vi "ExportPacketToCSV.vi"(6 "DefaultFolderName(Data)":string="Data", 7 "Prompt":string, 8 "Comment":string, 9 "NumerOfSamplesForAxis":i32, 10 "GyroData":waveform(dbl)[](array[waveform]), 11 "AccelData":waveform(dbl)[](array[waveform])) -> (0 "ErrorOut":errorcluster, 1 "Exported?":bool)   [LabVIEW 2016]
uses:
  <vilib>/Utility/file.llb/Write Delimited Spreadsheet (string).vi
  <vilib>/Utility/file.llb/Write Delimited Spreadsheet (DBL).vi
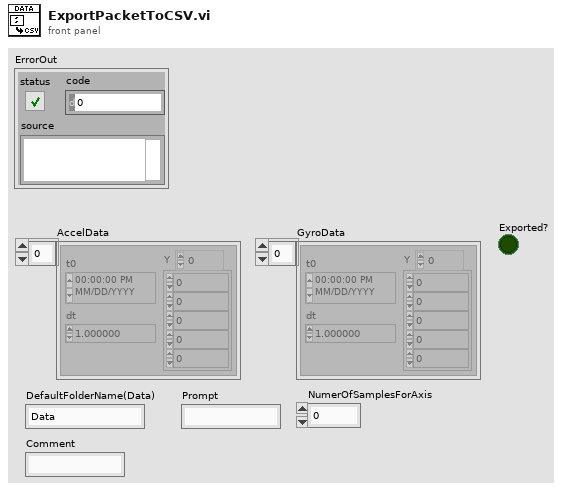
[diagram p1: front panel]
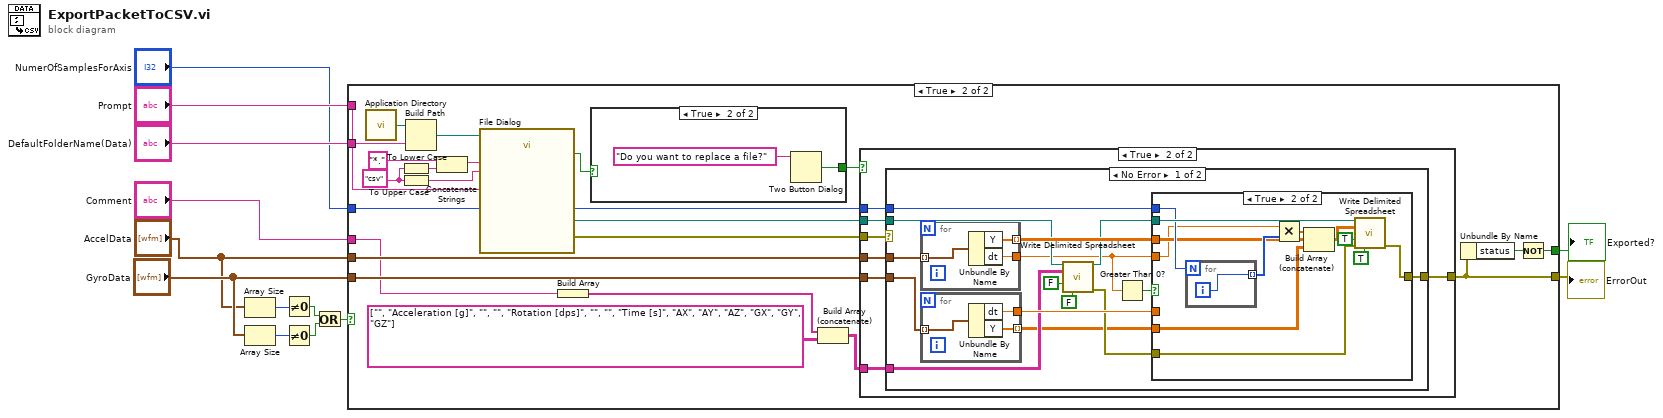
[diagram p0: block diagram]
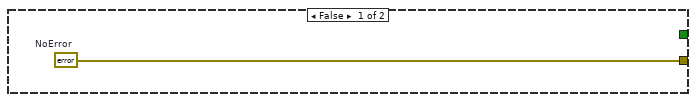
[diagram p2: hidden frame]
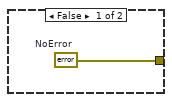
[diagram p3: hidden frame]
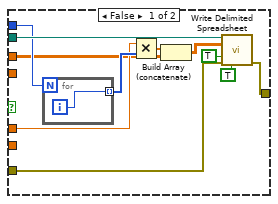
[diagram p4: hidden frame]
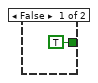
[diagram p6: hidden frame]
diagram:
  n1 = Array Size(array="AccelData") -> (size(s)=w8:i32)
  n2 = Array Size(array="GyroData") -> (size(s)=w9:i32)
  n3 = Not Equal To 0?(x=w8) -> (x != 0?=w6:bool)
  n4 = Not Equal To 0?(x=w9) -> (x != 0?=w5:bool)
  n5 = Or(x=w6, y=w5) -> (x .or. y?=w4:bool)
  n6 = case shown="True" w4 {
    tunnel: "DefaultFolderName(Data)" -> [_ w37]
    tunnel: [w14 w21] -> w12
    tunnel: "Prompt" -> [_ w36]
    tunnel: "GyroData" -> [_ w25]
    tunnel: "AccelData" -> [_ w24]
    tunnel: "NumerOfSamplesForAxis" -> [_ w22]
    tunnel: [_ w19] -> w2
    tunnel: "Comment" -> [_ w16]
    frame False {
      w14 = errorcluster {"status"=FALSE, "code"=0, "source"=""}  # NoError
    }
    frame True {
      w27 = "csv" ("string")
      n7 = call <vilib>:"Application Directory.vi"() -> ("Application Directory"=w35:path)
      n8 = To Lower Case(string=w27) -> (all lower case string=w32:string)
      n9 = To Upper Case(1:w27) -> (0:w33:string)
      n10 = Build Path(base path=w35, name or relative path=w37) -> (appended path=w34:path)
      n11 = Concatenate Strings("*." ("string"), w32) -> (w30:string)
      n12 = call "File Dialog"("start path"=w34, "prompt"=w36, "pattern (all files)"=w30, "pattern label"=w33) -> ("selected path"=w29:path, "exists"=w26:bool, "error out"=w28:errorcluster)  [unwired: 8 in, 1 out]
      n13 = Build Array(w16) -> (w15:string[])
      n14 = case shown="True" w26 {
        tunnel: [TRUE ("T button?") w95] -> w23
        frame False {
        }
        frame True {
          n15 = Two Button Dialog(message="Do you want to replace a file?") -> (T button?=w95:bool)  [unwired: 2 in]
        }
      }
      n16 = Build Array (concatenate)(w15, string[][] [["", "Acceleration [g]", "", "", "Rotation [dps]", "", ""], ["Time [s]", "AX", "AY", "AZ", "GX", "GY", "GZ"]]) -> (w18:string[][])
      n17 = case shown="True" w23 {
        tunnel: [w38 w45] -> w21
        tunnel: w29 -> [_ w44]
        tunnel: w28 -> [_ w43]
        tunnel: w24 -> [_ w42]
        tunnel: w25 -> [_ w41]
        tunnel: w22 -> [_ w40]
        tunnel: w18 -> [_ w39]
        frame False {
          w38 = errorcluster {"status"=FALSE, "code"=0, "source"=""}  # NoError
        }
        frame True {
          n18 = case shown="No Error" w43 {
            selector: w43 -> [_ w92]
            tunnel: [w55 w92] -> w45
            tunnel: w44 -> [w51 _]
            tunnel: w42 -> [w60 _]
            tunnel: w41 -> [w59 _]
            tunnel: w40 -> [w54 _]
            tunnel: w39 -> [w52 _]
            frame No Error {
              n19 = for {
                tunnel: w60 -> [w91] mode=indexing
                tunnel: [w90] -> w47
                tunnel: [w89] -> w56 mode=indexing
                n20 = Unbundle By Name(w91) -> ("Y"=w89:dbl[], "dt"=w90:dbl)
              }
              n21 = for {
                tunnel: w59 -> [w88] mode=indexing
                tunnel: [w87] -> w46 mode=indexing
                tunnel: [w86] -> w57
                n22 = Unbundle By Name(w88) -> ("dt"=w86:dbl, "Y"=w87:dbl[])
              }
              n23 = call-poly <vilib>:"Write Delimited Spreadsheet.vi"("file path (dialog if empty)"=w51, "2D data"=w52, "append to file? (new file:F)"=FALSE, "transpose? (no:F)"=FALSE) -> ("new file path (Not A Path if cancelled)"=w49:path, "error out"=w50:errorcluster)  [unwired: 10 in]
              n24 = Greater Than 0?(x=w47) -> (x > 0?=w58:bool)
              n25 = case shown="True" w58 {
                tunnel: w57 -> [w67 _]
                tunnel: w47 -> [_ w76]
                tunnel: w56 -> [w63 w77]
                tunnel: w49 -> [w70 w83]
                tunnel: [w66 w80] -> w55
                tunnel: w54 -> [w69 w82]
                tunnel: w50 -> [w62 w75]
                tunnel: w46 -> [_ w73]
                frame False {
                  n26 = for {
                    N: w69 -> [_]
                    tunnel: [w72] -> w68 mode=indexing
                    i -> [w72]
                  }
                  n27 = Multiply(x=w67, y=w68) -> (x*y=w64:dbl[])
                  n28 = Build Array (concatenate)(w64, w63) -> (w65:dbl[][])
                  n29 = call-poly <vilib>:"Write Delimited Spreadsheet.vi"("file path (dialog if empty)"=w70, "2D data"=w65, "append to file? (new file:F)"=TRUE, "error in (no error)"=w62, "transpose? (no:F)"=TRUE) -> ("error out"=w66:errorcluster)  [unwired: 9 in, 1 out]
                }
                frame True {
                  n30 = for {
                    N: w82 -> [_]
                    tunnel: [w85] -> w81 mode=indexing
                    i -> [w85]
                  }
                  n31 = Multiply(x=w76, y=w81) -> (x*y=w78:dbl[])
                  n32 = Build Array (concatenate)(w78, w77, w73) -> (w79:dbl[][])
                  n33 = call-poly <vilib>:"Write Delimited Spreadsheet.vi"("file path (dialog if empty)"=w83, "2D data"=w79, "append to file? (new file:F)"=TRUE, "error in (no error)"=w75, "transpose? (no:F)"=TRUE) -> ("error out"=w80:errorcluster)  [unwired: 9 in, 1 out]
                }
              }
            }
            frame Error {
            }
          }
        }
      }
      n34 = Unbundle By Name(w21) -> ("status"=w20:bool)
      n35 = Not(x=w20) -> (.not. x?=w19:bool)
    }
  }
  "ErrorOut" <- w12
  "Exported?" <- w2
